vi "GetFilePathFromRefnum.vi"(8 "error in (no error)":errorcluster, 11 "storage refnum":refnum<k20>) -> (0 "error out":errorcluster, 2 "storage location":path, 3 "storage refnum out":refnum<k20>)   [LabVIEW 2017]
uses:
  <resource>/objmgr/Storage.rc
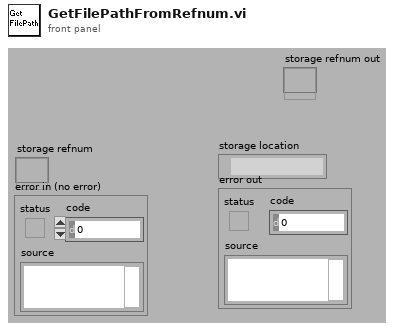
[diagram p1: front panel]
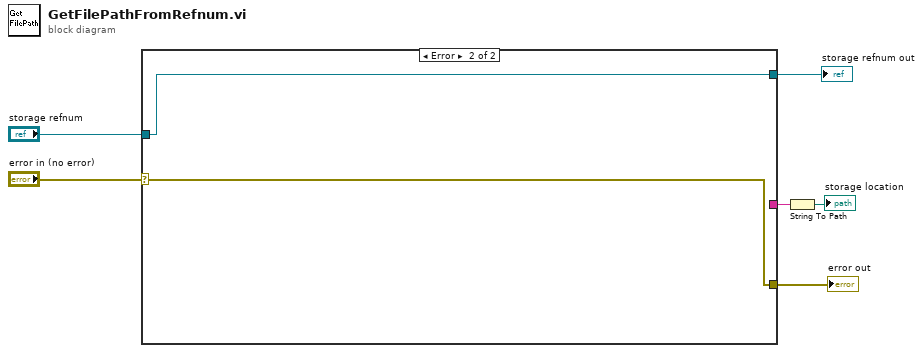
[diagram p0: block diagram]
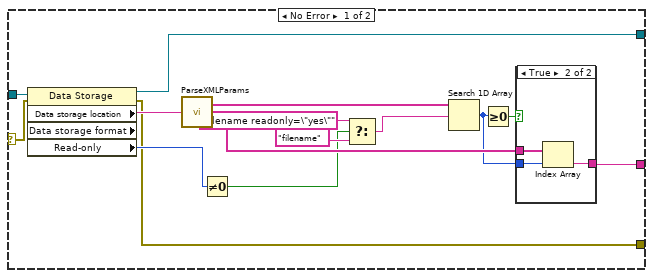
[diagram p2: hidden frame]
diagram:
  n1 = case shown="Error" "error in (no error)" {
    selector: "error in (no error)" -> [w8 w26]
    tunnel: "storage refnum" -> [w14 w25]
    tunnel: [w10 _] -> w4
    tunnel: [w9 w26] -> w3
    tunnel: [w7 w25] -> w1
    frame No Error {
      n2 = property class="Data Storage" props=["Data storage location", "Data storage format", "Read-only"](reference=w14, error in=w8) -> (reference out=w7:refnum<k20>, error out=w9:errorcluster, "Data storage location"=w13:string, "Read-only"=w12:i32)  [unwired: 1 out]
      n3 = call <vilib>:"ParseXMLParams.vi"("Parameter String"=w13) -> ("Names"=w21:string[], "Values"=w19:string[])
      n4 = Not Equal To 0?(x=w12) -> (x != 0?=w11:bool)
      n5 = Select(t="filename readonly=\"yes\"", s=w11, f="filename" ("element")) -> (s? t:f=w15:string)
      n6 = Search 1D Array(1D array=w21, element=w15) -> (index of element=w18:i32)  [unwired: 1 out]
      n7 = Greater Or Equal To 0?(x=w18) -> (x >= 0?=w20:bool)
      n8 = case shown="True" w20 {
        tunnel: w19 -> [_ w24]
        tunnel: w18 -> [_ w23]
        tunnel: [_ w22] -> w10
        frame False {
        }
        frame True {
          n9 = Index Array(array=w24, index=w23) -> (element=w22:string)
        }
      }
    }
    frame Error {
    }
  }
  "error out" <- w3
  "storage refnum out" <- w1
  n10 = String To Path(string=w4) -> (path=→"storage location":path)
